vi "20211008_HW03.vi"() -> ()   [LabVIEW 2019]
uses:
  <vilib>/Utility/miscctls.llb/LVBoundsTypeDef.ctl
panel:
  in  "Button":bool
  in  "Smaller":bool
  in  "Bigger":bool
  in  "Add Button Size":T1={"Width"=10, "Height"=10}
  in  "Button Size":T1={"Width"=50, "Height"=50}
  # "Press \"Page Up\" or \"Page Down\" key to change button size."
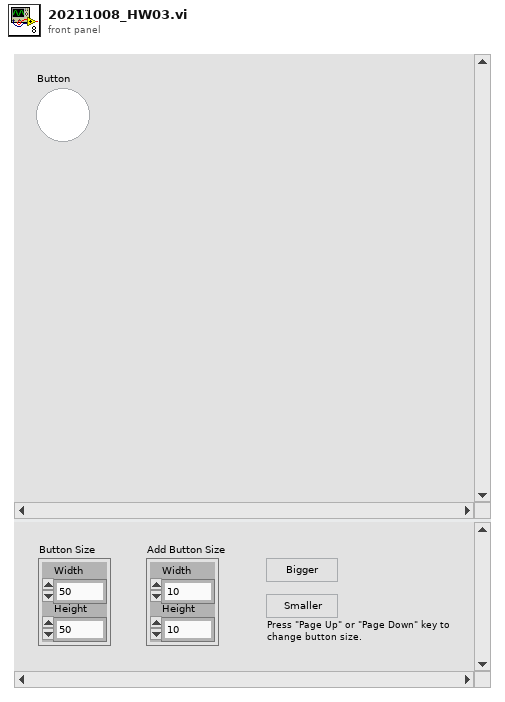
[diagram p1: front panel]
types:
  T1 = typedef "LVBoundsTypeDef.ctl" = cluster{"Width":u32, "Height":u32}
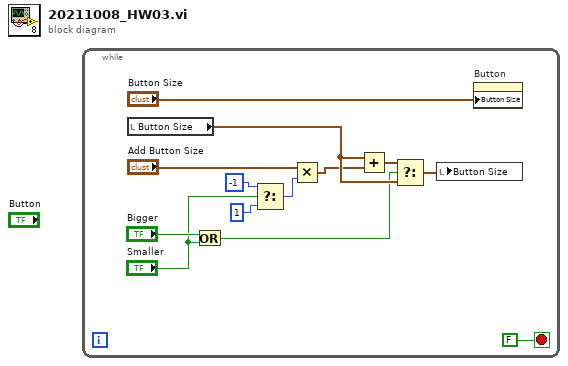
[diagram p0: block diagram]
diagram:
  n1 = while {
    stop <- FALSE stop-if-true
    n2 = local read "Button Size"() -> (w9:T1)
    n3 = Or(x="Bigger", y="Smaller") -> (x .or. y?=w5:bool)
    n4 = Select(t=-1, s="Smaller", f=1 ("t")) -> (s? t:f=w4:i32)
    n5 = Multiply(x="Add Button Size", y=w4) -> (x*y=w6:T1)
    n6 = Add(x=w9, y=w6) -> (x+y=w13:T1)
    n7 = Select(t=w13, s=w5, f=w9) -> (s? t:f=w10:T1)
    n8 = local write "Button Size"(w10) -> ()
    n9 = property on="Button" class="Bool"("Button Size"="Button Size") -> ()  [unwired: 2 in, 2 out]
  }
